vi "Execute Start Sequence.vi"(8 "error in (no error)":errorcluster, 10 "parameters":T1, 11 "Sequencer Module runtime in":refnum<class "Sequencer Module runtime.lvclass">) -> (0 "error out":errorcluster, 2 "Parameters allocation out":T1, 3 "Sequencer Module runtime out":refnum<class "Sequencer Module runtime.lvclass">)   [LabVIEW 2015, in "Sequencer Module runtime.lvclass"]
uses:
  Sequencer Module runtime.lvclass
  <vilib>/NI/Tag Bus/table/data table.ctl
  Sequencer State Enum.ctl
  classes/Step/Execution/StepState.ctl
  classes/Step/Execution/Step Status.ctl
  classes/Step/Execution/Step Flow Control.ctl
  Sequencer Module runtime.lvclass/Sequencer Module runtime.ctl
  classes/Results List/Results List.lvclass
  classes/Step/Execution/Step.lvclass
  classes/Sequence/Execution/Sequence.lvclass
  <vilib>/NI/Tag Bus/table/data table.lvlib
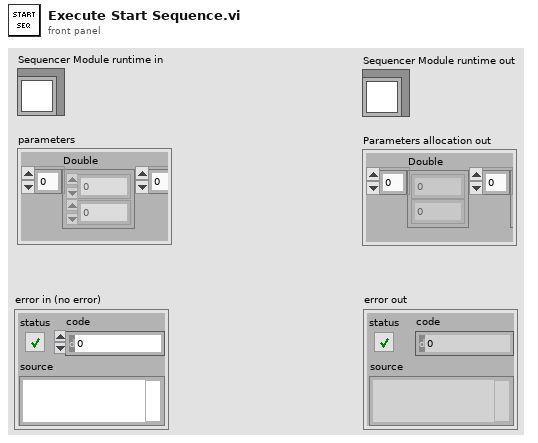
[diagram p1: front panel]
types:
  T1 = typedef "tag bus.lvlib/data table.lvlib/data table.ctl" = cluster{"Double":dbl[], "Single":sgl[], "I64":i64[], "I32":i32[], "I16":i16[], "I8":i8[], "U64":u64[], "U32":u32[], "U16":u16[], "U8":u8[], "Boolean":bool[], "String":string[], "Array of Double":cluster{"DBL Array":dbl[]}[], "Array of Single":cluster{"SGL Array":sgl[]}[], "Array of I64":cluster{"I64 Array":i64[]}[], "Array of I32":cluster{"I32 Array":i32[]}[], "Array of I16":cluster{"I16 Array":i16[]}[], "Array of I8":cluster{"I8 Array":i8[]}[], "Array of U64":cluster{"U64 Array":u64[]}[], "Array of U32":cluster{"U32 Array":u32[]}[], "Array of U16":cluster{"U16 Array":u16[]}[], "Array of U8":cluster{"U8 Array":u8[]}[], "Array of Boolean":cluster{"Boolean Array":bool[]}[], "Array of String":cluster{"String Array":string[]}[]}
  T2 = typedef "Step.lvclass/StepState.ctl" = cluster{"Step State":T3, "Flow Control":T4, "Jump Index":i32, "Done":bool}
  T3 = typedef "Step.lvclass/Step Status.ctl" = enum16{"Start", "Passed", "Failed", "Error", "Done", "Terminated", "Skipped", "Running"}
  T4 = typedef "Step.lvclass/Step Flow Control.ctl" = enum16{"Next Step", "Jump"}
  T5 = typedef "Sequencer Module runtime.lvclass/Sequencer State Enum.ctl" = enum16{"Idle", "Paused", "Start Sequence", "Run Sequence", "CleanUp Sequence", "Generate Report"}
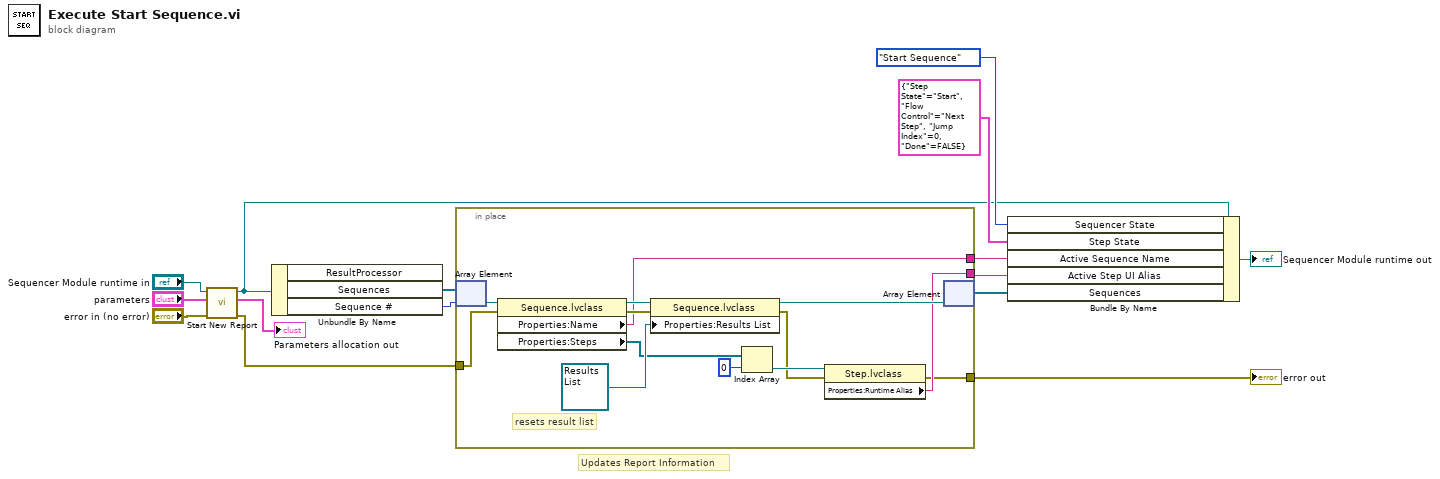
[diagram p0: block diagram]
diagram:
  # "Updates Report Information"
  n1 = call "Start New Report.vi"("error in (no error)"="error in (no error)", "parameters"="parameters", "Sequencer Module runtime in"="Sequencer Module runtime in") -> ("error out"=w1:errorcluster, "Parameters allocation out"=→"Parameters allocation out":T1, "Sequencer Module runtime out"=w2:refnum<class "Sequencer Module runtime.lvclass">)  [unwired: 6 in]
  n2 = Unbundle By Name(w2) -> ("Sequences"=w12:refnum<class "Sequence.lvclass">[], "Sequence #"=w11:i32)  [unwired: 1 out]
  n3 = in-place {
    in-place-border: [w20] -> w9
    in-place-border: [w18] -> w8
    in-place-border: w1 -> [w19]
    in-place-border: [w16] -> w7
    # "resets result list"
    n4 = in-place-array #1(w12, w11) -> (w26:refnum<class "Sequence.lvclass">)
    n5 = property class="Sequence.lvclass"(reference=w26, error in=w19) -> (reference out=w25:refnum<class "Sequence.lvclass">, error out=w24:errorcluster, "Properties:Name"=w20:string, "Properties:Steps"=w21:refnum<class "Step.lvclass">[])
    n6 = property class="Sequence.lvclass"(reference=w25, error in=w24, "Properties:Results List"=refnum<class "Results List.lvclass"> refnum ("Results List")) -> (reference out=w27:refnum<class "Sequence.lvclass">, error out=w17:errorcluster)
    n7 = Index Array(array=w21, index=0 ("Sequencer State.Active Step")) -> (element=w23:refnum<class "Step.lvclass">)
    n8 = property class="Step.lvclass"(reference=w23, error in=w17) -> (error out=w16:errorcluster, "Properties:Runtime Alias"=w18:string)  [unwired: 1 out]
    n9 = in-place-array #1(w27) -> (w10:refnum<class "Sequence.lvclass">[])  [unwired: 1 out]
  }
  "error out" <- w7
  n10 = Bundle By Name(cluster=w2, "Sequencer State"=Sequencer_State_Enum."Start Sequence" ("Sequencer State.Sequencer State"), "Step State"=T2 {"Step State"=enum."Start", "Flow Control"=enum."Next Step", "Jump Index"=0, "Done"=FALSE} ("Sequencer State.Step State"), "Active Sequence Name"=w9, "Active Step UI Alias"=w8, "Sequences"=w10) -> (→"Sequencer Module runtime out":refnum<class "Sequencer Module runtime.lvclass">)
